vi "ETPA&SPIRTONE PROGRAM V1.vi"() -> ()   [LabVIEW 2024]
uses:
  <vilib>/Instr/_visa.llb/VISA Find Search Mode.ctl
  <vilib>/Instr/_visa.llb/VISA Open Access Mode.ctl
panel:
  in  "PMT counts for average":i32
  out "PMT counts for average":i32
  out "PRESENT MULTIMETER AVERAGE":dbl(graph)
  out "multimeter counts for average":i32
  in  "multimeter counts for average":i32
  out "Multimeter Connecteion status":string
  out "error out 2":errorcluster
  in  "error in (no error)":errorcluster
  out "Monochromator Connecteion status":string
  in  "Close Shutter":bool
  in  "Open Shutter":bool
  out "PRESENT - COUNTER Averaged":dbl(graph)
  in  "Number of Measuments per average PMT WAVESCAN":i32
  out "Number of Measuments per average PMT WAVESCAN":i32
  in  "Monochromator":refnum<visa-resource-name>
  in  "Step Size (nm)":dbl
  in  "End W/L (nm)":dbl
  in  "Start W/L (nm)":dbl
  out "Present Monochromator":dbl(graph)
  out "SHUTTER STATUS":string="SHUTTER O"
  in  "Go scan":bool
  in  "Stop WAVE":bool
  in  "number of measurements":i32
  out "number of measurements":i32
  out "break time ms 2":u32=100
  out "Collection Time 2":u32=1000
  out "Function (1: AC Volts)\nFunction(0: DC Volts)":u16=1
  out "counter  2":tag="Dev1/ctr0"
  out "source  2":tag="/Dev1/PFI14"
  in  "VISA resource name mulitmeter":refnum<visa-resource-name>
  in  "DEFAULT?":bool
  in  "Collection Time":u32
  in  "Label?":bool
  in  "Wavescan?":bool
  in  "file path (dialog if empty)":path
  in  "?":bool
  out "PRESENT - COUNTER":dbl(graph)
  out "PRESENT - Multimeter":dbl(graph)
  in  "Function (1: AC Volts)\nFunction(0: DC Volts)":u16
  in  "break time ms":u32
  in  "source":tag
  in  "counter":tag
  out "Current Trial -Multimeter":dbl(graph)
  out "Current Trial - Singles Photon Count Rate":dbl(graph)
  in  "speed of taking measurments":u32
  # "Default Settings"
  # "CTR0"
  # "USB0"
  # "PFI14"
  # "Not Default Settings"
  # "PLEASE PUT (\".csv\") at the end of your path"
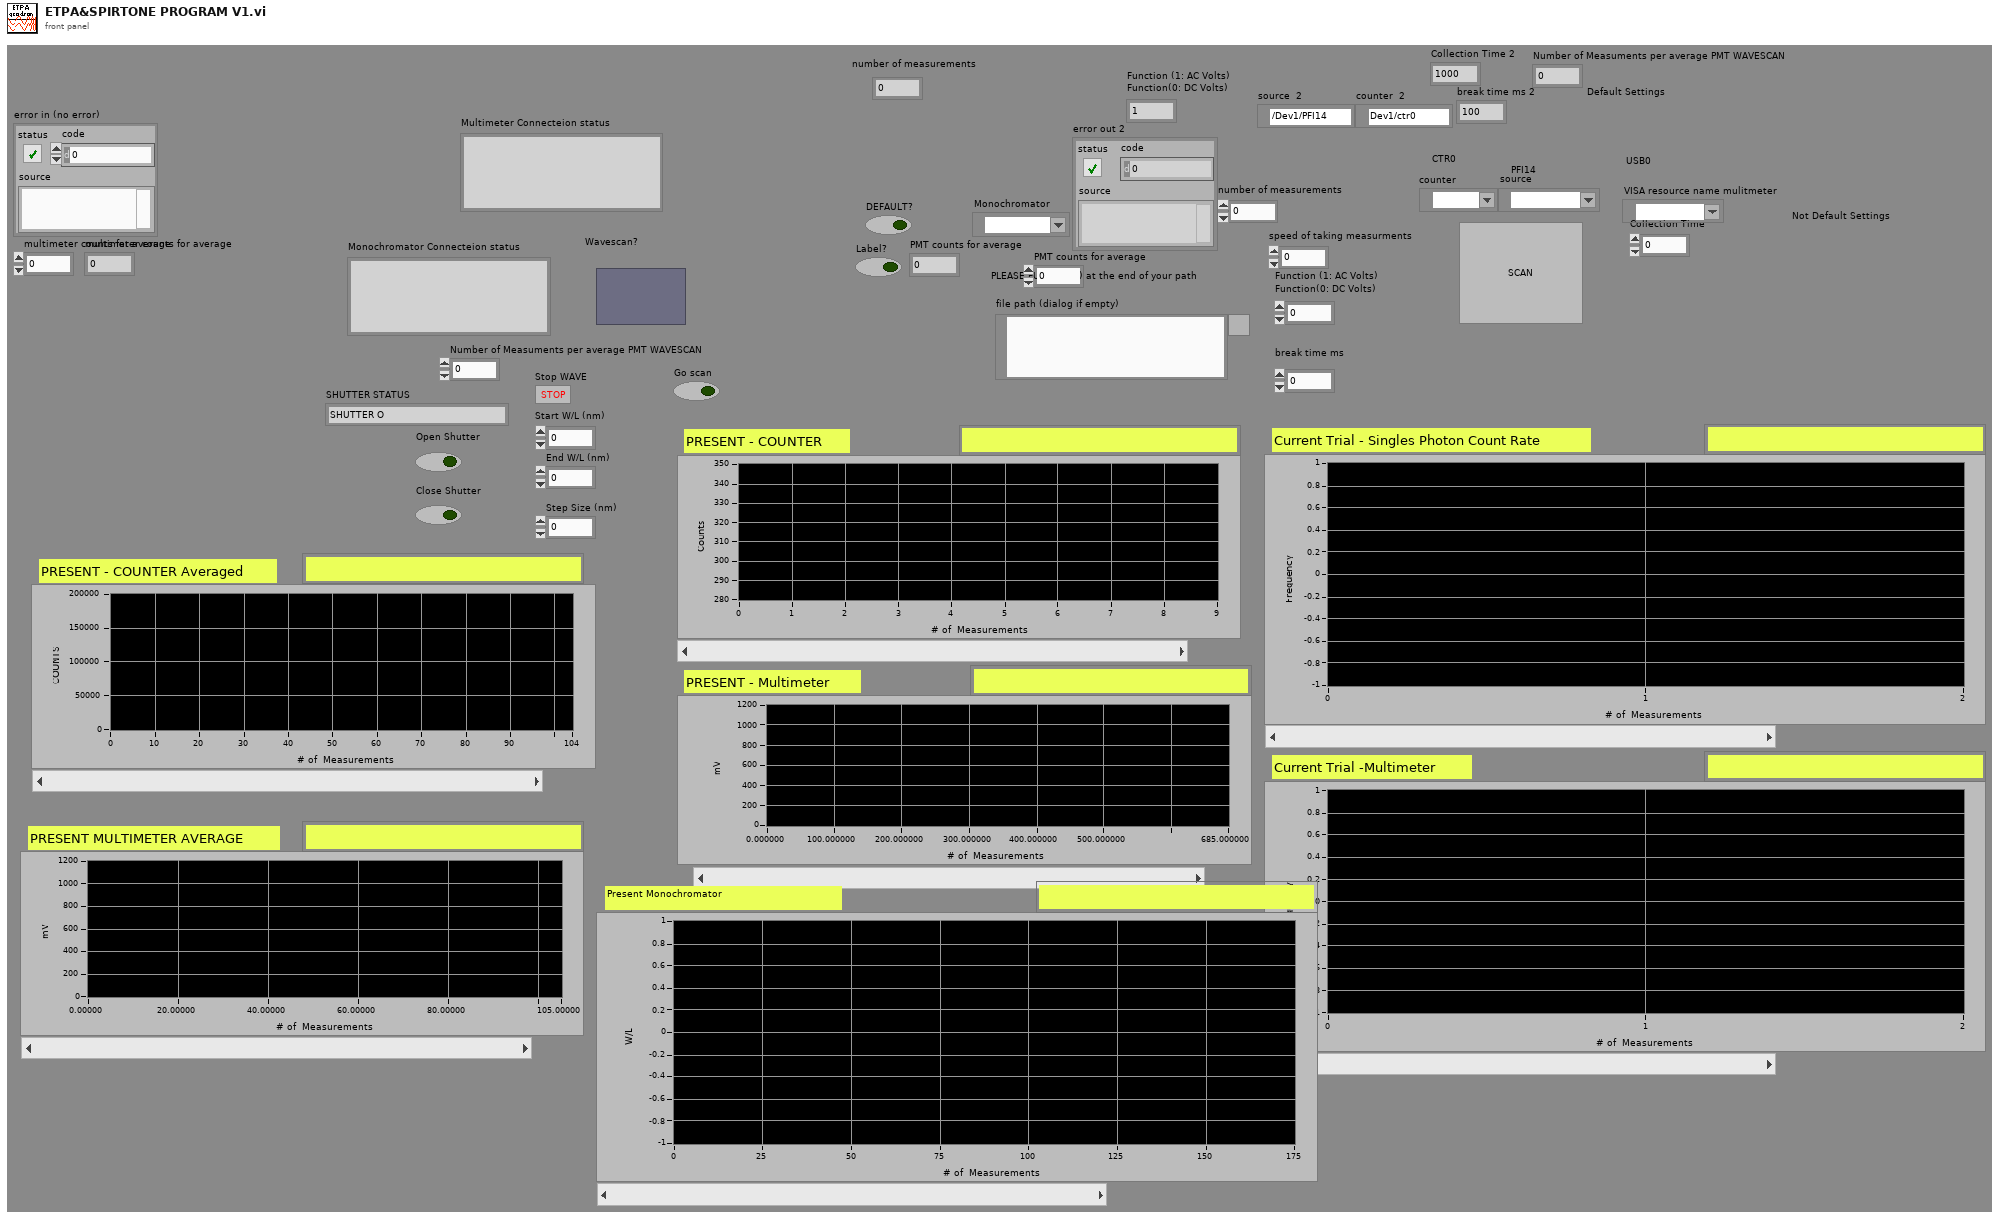
[diagram p1: front panel]
types:
  T1 = typedef "VISA Find Search Mode.ctl" = u32
  T2 = typedef "VISA Open Access Mode.ctl" = u32
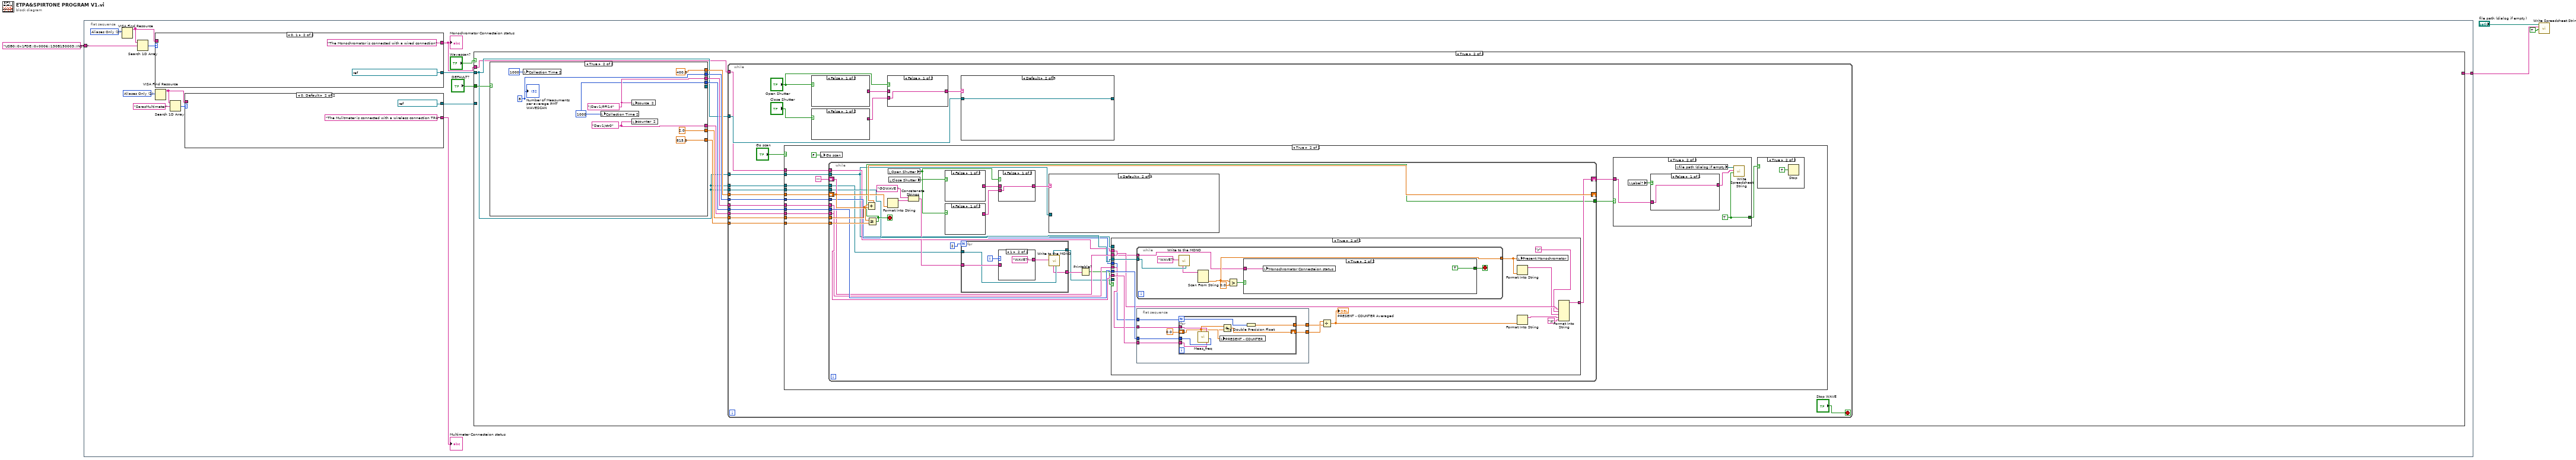
[diagram p0: block diagram]
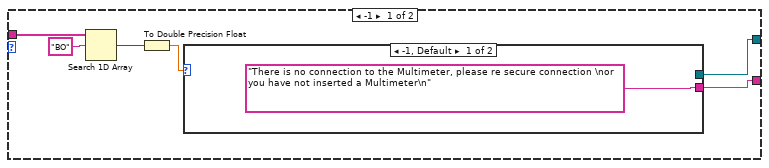
[diagram p2: hidden frame]
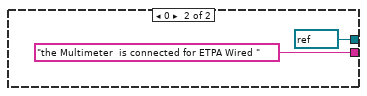
[diagram p3: hidden frame]
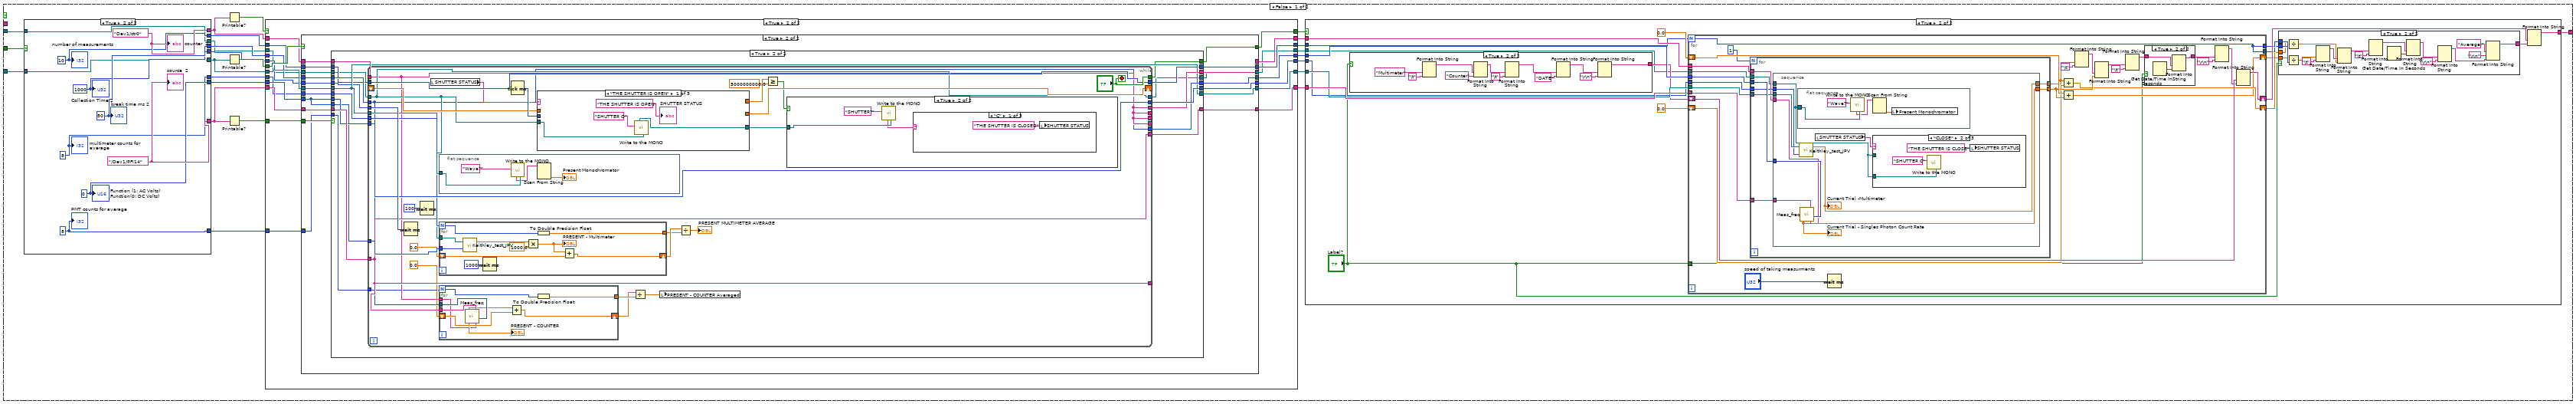
[diagram p4: hidden frame]
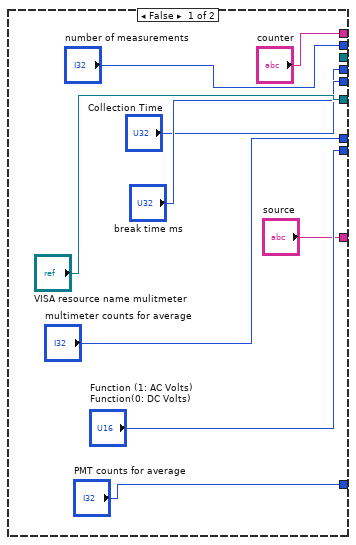
[diagram p5: hidden frame]
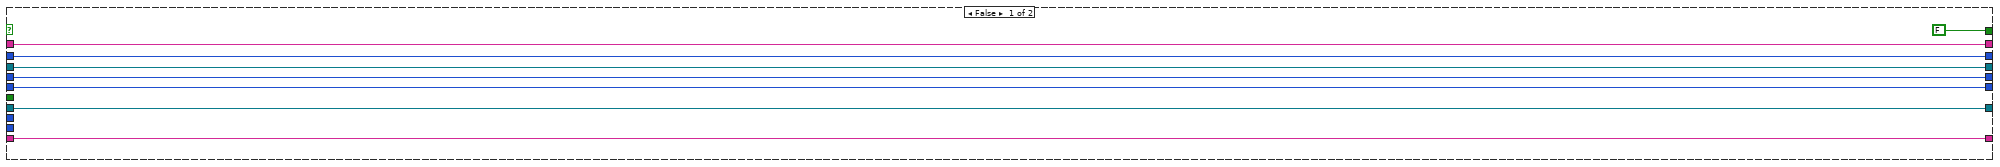
[diagram p6: hidden frame]
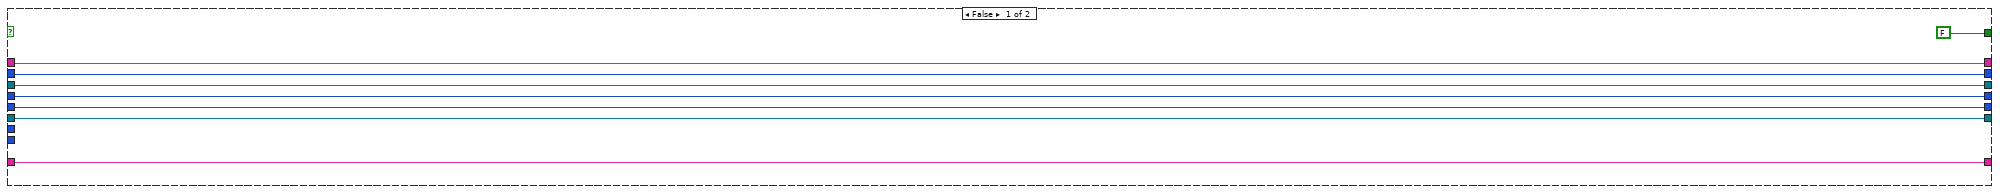
[diagram p7: hidden frame]
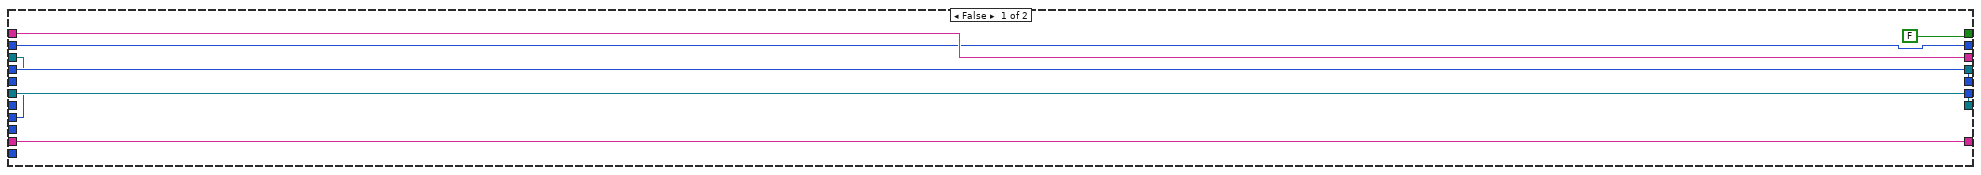
[diagram p8: hidden frame]
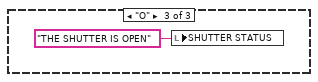
[diagram p11: hidden frame]
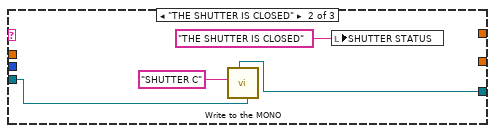
[diagram p12: hidden frame]
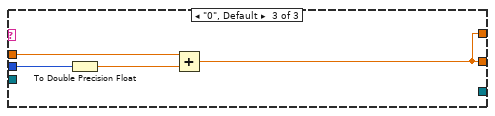
[diagram p13: hidden frame]
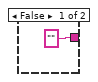
[diagram p14: hidden frame]
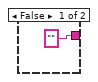
[diagram p15: hidden frame]
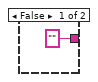
[diagram p16: hidden frame]
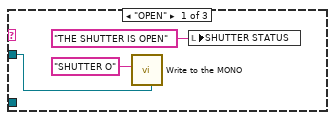
[diagram p18: hidden frame]
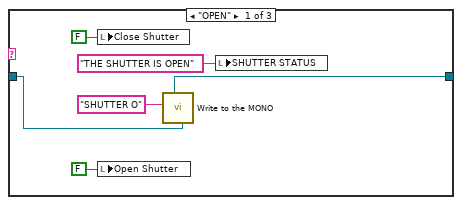
[diagram p20: hidden frame]
diagram:
  n1 = flat-sequence {
    tunnel: [w17] -> w2
    tunnel: "USB0::0x1FDE::0x0006::130B150003::INSTR" ("element") -> [w13]
    frame #0 {
      w10 = T1 2 items=["Canonical Names Only"=0, "Aliases Only"=2, "Include Matching Aliases"=3, "Include All Aliases"=4] ("Search Mode")
      w16 = T1 2 items=["Canonical Names Only"=0, "Aliases Only"=2, "Include Matching Aliases"=3, "Include All Aliases"=4] ("Search Mode")
      n2 = VISA Find Resource(10:w16) -> (3:w15:string[])  [unwired: 2 in, 2 out]
      n3 = Search 1D Array(1D array=w15, element=w13) -> (index of element=w12:i32)  [unwired: 1 in]
      n4 = case shown="0, 1" w12 {
        tunnel: [w523 refnum<visa-resource-name> "USB0::0x1FDE::0x0006::130B150003::INSTR" ("VISA resource name mulitmeter")] -> w14
        tunnel: w15 -> [w525 _]
        tunnel: [w522 "The Monochromator is connected with a wired connection"] -> w11
        frame -1, Default {
          n5 = Search 1D Array(1D array=w525, element="remote130Bmonochromator") -> (index of element=w521:i32)  [unwired: 1 in]
          n6 = To Double Precision Float(number=w521) -> (double precision float=w520:dbl)
          n7 = case shown="-1, Default" w520 {
            tunnel: [_ refnum<visa-resource-name> "USB0::0x1FDE::0x0006::130B150003::INSTR" ("VISA resource name mulitmeter")] -> w523
            tunnel: ["There is no connection to the monochromator, please re secure connection \nor you have not inserted a 130B cornerstone monochromator\n" "the Monochromator is connected romotely"] -> w522
            frame -1, Default {
            }
            frame 0..3 {
            }
          }
        }
        frame 0, 1 {
        }
      }
      "Monochromator Connecteion status" <- w11
      n8 = VISA Find Resource(10:w10) -> (3:w9:string[])  [unwired: 2 in, 2 out]
      n9 = Search 1D Array(1D array=w9, element="SarasMultimeter") -> (index of element=w7:i32)  [unwired: 1 in]
      n10 = case shown="0, Default" w7 {
        tunnel: [w23 refnum<visa-resource-name> "sarasMultimeter" ("VISA resource name mulitmeter")] -> w5
        tunnel: w9 -> [w25 _]
        tunnel: [w22 "The Mulitmeter is connected with a wireless connection TPA"] -> w6
        frame -1 {
          n11 = Search 1D Array(1D array=w25, element="BO") -> (index of element=w21:i32)  [unwired: 1 in]
          n12 = To Double Precision Float(number=w21) -> (double precision float=w20:dbl)
          n13 = case shown="-1, Default" w20 {
            tunnel: [_ refnum<visa-resource-name> "BO" ("VISA resource name mulitmeter")] -> w23
            tunnel: ["There is no connection to the Multimeter, please re secure connection \nor you have not inserted a Multimeter\n" "the Multimeter  is connected for ETPA Wired "] -> w22
            frame -1, Default {
            }
            frame 0 {
            }
          }
        }
        frame 0, Default {
        }
      }
      "Multimeter Connecteion status" <- w6
      n14 = case shown="True" "Wavescan?" {
        tunnel: "DEFAULT?" -> [w40 w340]
        tunnel: [w35 _] -> w17
        tunnel: w14 -> [w34 w332]
        tunnel: w11 -> [_ w331]
        tunnel: w5 -> [w33 _]
        frame False {
          n15 = case shown="True" w40 {
            tunnel: ["VISA resource name mulitmeter" w68] -> w46
            tunnel: ["break time ms" w74] -> w45
            tunnel: ["Collection Time" w73] -> w44
            tunnel: ["Function (1: AC Volts)\nFunction(0: DC Volts)" w67] -> w43
            tunnel: ["source" w72] -> w42
            tunnel: ["counter" w71] -> w41
            tunnel: ["number of measurements" w70] -> w38
            tunnel: [_ w69] -> w37
            tunnel: w34 -> [_ w69]
            tunnel: w33 -> [_ w68]
            tunnel: ["multimeter counts for average" w66] -> w32
            tunnel: ["PMT counts for average" w65] -> w31
            frame False {
            }
            frame True {
              w65 = 8 ("PMT counts for average")
              w66 = 8 ("Numeric 2")
              w67 = u16 0 ("Function (1: AC Volts)\nFunction(0: DC Volts)")
              w70 = 10
              w71 = tag "Dev1/ctr0" ("counter")
              w72 = tag "/Dev1/PFI14" ("source")
              w73 = u32 1000 ("Collection Time")
              w74 = u32 50 ("break time ms")
              "source  2" <- w72
              "counter  2" <- w71
              "Function (1: AC Volts)\nFunction(0: DC Volts)" <- w67
              "Collection Time 2" <- w73
              "break time ms 2" <- w74
              "number of measurements" <- w70
              "multimeter counts for average" <- w66
              "PMT counts for average" <- w65
            }
          }
          n16 = Printable?(1:w41) -> (0:w49:bool)
          n17 = Printable?(1:w46) -> (0:w48:bool)
          n18 = Printable?(1:w42) -> (0:w47:bool)
          n19 = case shown="True" w49 {
            tunnel: w48 -> [_ w102]
            tunnel: w47 -> [_ w101]
            tunnel: w41 -> [w80 w100]
            tunnel: w46 -> [w78 w99]
            tunnel: w42 -> [w81 w98]
            tunnel: w45 -> [w79 w97]
            tunnel: w43 -> [_ w96]
            tunnel: [w81 w95] -> w55
            tunnel: [w78 w94] -> w54
            tunnel: [w79 w93] -> w53
            tunnel: [w80 w92] -> w52
            tunnel: [FALSE w91] -> w51
            tunnel: [w77 w90] -> w50
            tunnel: w44 -> [w77 w89]
            tunnel: w38 -> [w76 w88]
            tunnel: [w76 w87] -> w39
            tunnel: w37 -> [w75 w86]
            tunnel: [w75 w85] -> w36
            tunnel: w32 -> [_ w84]
            tunnel: w31 -> [_ w83]
            frame False {
            }
            frame True {
              n20 = case shown="True" w102 {
                tunnel: w101 -> [_ w129]
                tunnel: w100 -> [w108 w128]
                tunnel: w99 -> [w107 w113]
                tunnel: w98 -> [w110 w127]
                tunnel: w97 -> [w109 w126]
                tunnel: w96 -> [_ w125]
                tunnel: [w110 w124] -> w95
                tunnel: [w107 w123] -> w94
                tunnel: [w109 w122] -> w93
                tunnel: [w108 w121] -> w92
                tunnel: [FALSE w120] -> w91
                tunnel: [w105 w119] -> w90
                tunnel: w89 -> [w105 w118]
                tunnel: w88 -> [w104 w117]
                tunnel: [w104 w116] -> w87
                tunnel: w86 -> [w103 w115]
                tunnel: [w103 w114] -> w85
                tunnel: w84 -> [_ w112]
                tunnel: w83 -> [_ w111]
                frame False {
                }
                frame True {
                  n21 = case shown="True" w129 {
                    tunnel: [w136 w150] -> w124
                    tunnel: [w137 w149] -> w123
                    tunnel: [w134 w153] -> w122
                    tunnel: [w135 w151] -> w121
                    tunnel: [FALSE w148] -> w120
                    tunnel: [w132 w152] -> w119
                    tunnel: w128 -> [w135 w154]
                    tunnel: w113 -> [w137 w149]
                    tunnel: w127 -> [w136 w155]
                    tunnel: w126 -> [_ w147]
                    tunnel: w125 -> [w134 w146]
                    tunnel: w125 -> [_ w145]
                    tunnel: w118 -> [w132 w144]
                    tunnel: w117 -> [w131 w143]
                    tunnel: [w131 w142] -> w116
                    tunnel: w115 -> [w130 w141]
                    tunnel: [w130 w140] -> w114
                    tunnel: w112 -> [_ w139]
                    tunnel: w111 -> [_ w138]
                    frame False {
                    }
                    frame True {
                      n22 = while {
                        tunnel: [w182] -> w153
                        tunnel: [w162] -> _
                        tunnel: [w161] -> w152
                        tunnel: [w162] -> _
                        tunnel: [w162] -> _
                        tunnel: [w163] -> _
                        tunnel: w149 -> [w166]
                        tunnel: w155 -> [w163]
                        tunnel: w154 -> [w162]
                        tunnel: [w162] -> w151
                        tunnel: [w163] -> w150
                        tunnel: ["?"] -> w148
                        tunnel: w147 -> [w183]
                        tunnel: w146 -> [w182]
                        tunnel: w145 -> [w165]
                        tunnel: w144 -> [w161]
                        tunnel: w143 -> [w181]
                        tunnel: [w181] -> w142
                        shift-right: [w178] -> _
                        shift-left: _ -> [w177]
                        tunnel: w141 -> [w172]
                        tunnel: [w172] -> w140
                        tunnel: w139 -> [w170]
                        tunnel: w138 -> [w158]
                        stop <- "?" stop-if-true
                        n23 = Wait (ms)(milliseconds to wait=w183) -> ()  [unwired: 1 out]
                        n24 = Wait (ms)(milliseconds to wait=u32 100) -> ()  [unwired: 1 out]
                        n25 = local read "SHUTTER STATUS"() -> (w171:string)
                        n26 = flat-sequence {
                          tunnel: w172 -> [w205]
                          frame #0 {
                            n27 = call "Write to the MONO.vi"("MONOCHOMATOR"=w205, "write buffer"="Wave?") -> ("read buffer"=w203:string)  [unwired: 7 in, 2 out]
                            n28 = Scan From String(input string=w203) -> (output 1=→"Present Monochromator":dbl)  [unwired: 4 in, 3 out]
                          }
                        }
                        n29 = for {
                          N: w170 -> [w202]
                          shift-right: [w200] -> w169
                          shift-left: 0.0 -> [w201]
                          tunnel: [w199] -> w168
                          tunnel: w166 -> [w198]
                          tunnel: w165 -> [w197]
                          n30 = call "Keithley_test_JPV.vi"("Function (0: DC Volts)"=w197, "VISA resource name"=w198) -> ("Measurement"=w195:dbl)  [unwired: 1 out]
                          n31 = Wait (ms)(milliseconds to wait=u32 1000) -> ()  [unwired: 1 out]
                          n32 = Multiply(x=w195, y=1000.0) -> (x*y=w193:dbl)
                          "PRESENT - Multimeter" <- w193
                          n33 = To Double Precision Float(number=w202) -> (double precision float=w199:dbl)
                          n34 = Add(x=w193, y=w201) -> (x+y=w200:dbl)
                        }
                        n35 = for {
                          N: w158 -> [w187]
                          tunnel: w163 -> [w192]
                          tunnel: w162 -> [w185]
                          tunnel: w161 -> [w191]
                          shift-right: [w188] -> w156
                          shift-left: 0.0 -> [w190]
                          tunnel: [w186] -> w157
                          n36 = call "Meas_freq.vi"("source"=w192, "Time miliseconds"=w191, "counter"=w185) -> (0:w189:dbl)  [unwired: 1 in]
                          "PRESENT - COUNTER" <- w189
                          n37 = Add(x=w189, y=w190) -> (x+y=w188:dbl)
                          n38 = To Double Precision Float(number=w187) -> (double precision float=w186:dbl)
                        }
                        n39 = Tick Count (ms)() -> (millisecond timer value=w179:u32)
                        n40 = case shown="\"THE SHUTTER IS OPEN\"" w171 {
                          tunnel: w179 -> [_ _ w221]
                          tunnel: [_ _ w222] -> w178
                          tunnel: w177 -> [_ _ w223]
                          tunnel: [_ _ w222] -> w175
                          tunnel: [w213 w217 _] -> w173
                          tunnel: w172 -> [w214 w218 _]
                          frame "THE SHUTTER IS OPEN" {
                            n41 = call "Write to the MONO.vi"("MONOCHOMATOR"=w214, "write buffer"="SHUTTER O") -> ("VISA resource name out"=w213:refnum<visa-resource-name>)  [unwired: 7 in, 2 out]
                            "SHUTTER STATUS" <- "THE SHUTTER IS OPEN" ("String")
                          }
                          frame "THE SHUTTER IS CLOSED" {
                            n42 = call "Write to the MONO.vi"("MONOCHOMATOR"=w218, "write buffer"="SHUTTER C") -> ("VISA resource name out"=w217:refnum<visa-resource-name>)  [unwired: 7 in, 2 out]
                            n43 = local write "SHUTTER STATUS"("THE SHUTTER IS CLOSED" ("String")) -> ()
                          }
                          frame "0", Default {
                            n44 = To Double Precision Float(number=w221) -> (double precision float=w220:dbl)
                            n45 = Add(x=w223, y=w220) -> (x+y=w222:dbl)
                          }
                        }
                        n46 = Divide(x=w156, y=w157) -> (x/y=w159:dbl)
                        n47 = local write "PRESENT - COUNTER Averaged"(w159) -> ()
                        n48 = Divide(x=w169, y=w168) -> (x/y=→"PRESENT MULTIMETER AVERAGE":dbl)
                        n49 = Greater Or Equal?(x=w175, y=5000000000.0) -> (x >= y?=w176:bool)
                        n50 = case shown="True" w176 {
                          tunnel: w173 -> [_ w209]
                          frame False {
                          }
                          frame True {
                            n51 = call "Write to the MONO.vi"("MONOCHOMATOR"=w209, "write buffer"="SHUTTER?") -> ("read buffer"=w207:string)  [unwired: 7 in, 2 out]
                            n52 = case shown="\"C\"" w207 {
                              frame "C" {
                                n53 = local write "SHUTTER STATUS"("THE SHUTTER IS CLOSED" ("SHUTTER STATUS")) -> ()
                              }
                              frame Default {
                              }
                              frame "O" {
                                n54 = local write "SHUTTER STATUS"("THE SHUTTER IS OPEN" ("SHUTTER STATUS")) -> ()
                              }
                            }
                          }
                        }
                      }
                    }
                  }
                }
              }
            }
          }
          n55 = case shown="True" w51 {
            tunnel: w50 -> [_ w242]
            tunnel: w55 -> [_ w241]
            tunnel: w54 -> [_ w240]
            tunnel: w53 -> [_ w239]
            tunnel: w52 -> [_ w238]
            tunnel: w39 -> [_ w227]
            tunnel: ["" w226] -> w35
            tunnel: w36 -> [_ w225]
            frame False {
            }
            frame True {
              n56 = case shown="True" "Label?" {
                tunnel: ["" w249] -> w237
                frame False {
                }
                frame True {
                  n57 = Format Into String("Multimeter" ("input 2"), "\t") -> (resulting string=w253:string)  [unwired: 3 in, 1 out]
                  n58 = Format Into String(w253, "Counter" ("input 2")) -> (resulting string=w248:string)  [unwired: 3 in, 1 out]
                  n59 = Format Into String(w248, "\t") -> (resulting string=w246:string)  [unwired: 3 in, 1 out]
                  n60 = Format Into String(w246, "DATE" ("input 2")) -> (resulting string=w245:string)  [unwired: 3 in, 1 out]
                  n61 = Format Into String(w245, "\r\n") -> (resulting string=w249:string)  [unwired: 3 in, 1 out]
                }
              }
              n62 = for {
                N: w227 -> [w292]
                tunnel: w242 -> [w299]
                tunnel: w241 -> [w298]
                tunnel: w240 -> [w297]
                tunnel: w239 -> [w296]
                tunnel: w238 -> [w295]
                shift-right: [w293] -> w236
                shift-left: w237 -> [w294]
                shift-right: [w277] -> w229
                shift-left: 0.0 -> [w282]
                shift-right: [w278] -> w231
                shift-left: 0.0 -> [w279]
                tunnel: [w292] -> w230
                tunnel: [w292] -> w232
                tunnel: "Label?" -> [w276]
                tunnel: w225 -> [w274]
                n63 = for {
                  N: 1 -> [_]
                  tunnel: w299 -> [w311]
                  tunnel: w298 -> [w310]
                  tunnel: w297 -> [w309]
                  tunnel: w296 -> [w308]
                  tunnel: w295 -> [w307]
                  tunnel: [w306] -> w280
                  tunnel: [w305] -> w281
                  tunnel: w274 -> [w304]
                  n64 = stacked-sequence {
                    tunnel: w311 -> [w320]
                    tunnel: w310 -> [w319]
                    tunnel: w309 -> [w318]
                    tunnel: w308 -> [w317]
                    tunnel: w307 -> [w312]
                    tunnel: [w316] -> w306
                    tunnel: [w315] -> w305
                    tunnel: w304 -> [w313]
                    frame #0 {
                      n65 = flat-sequence {
                        tunnel: w313 -> [w323]
                        frame #0 {
                          n66 = call "Write to the MONO.vi"("MONOCHOMATOR"=w323, "write buffer"="Wave?") -> ("read buffer"=w321:string)  [unwired: 7 in, 2 out]
                          n67 = Scan From String(input string=w321) -> (output 1=w324:dbl)  [unwired: 4 in, 3 out]
                          n68 = local write "Present Monochromator"(w324) -> ()
                        }
                      }
                      n69 = call "Keithley_test_JPV.vi"("Function (0: DC Volts)"=w317, "VISA resource name"=w318) -> ("Measurement"=w316:dbl)  [unwired: 1 out]
                      "Current Trial -Multimeter" <- w316
                      n70 = call "Meas_freq.vi"("source"=w319, "Time miliseconds"=w320, "counter"=w312) -> (0:w315:dbl)  [unwired: 1 in]
                      "Current Trial - Singles Photon Count Rate" <- w315
                      n71 = local read "SHUTTER STATUS"() -> (w314:string)
                      n72 = case shown="\"CLOSE\"" w314 {
                        tunnel: w313 -> [w326 _ _]
                        tunnel: w313 -> [_ w329 _]
                        frame "OPEN" {
                          n73 = call "Write to the MONO.vi"("MONOCHOMATOR"=w326, "write buffer"="SHUTTER O") -> ()  [unwired: 7 in, 3 out]
                          n74 = local write "SHUTTER STATUS"("THE SHUTTER IS OPEN" ("String")) -> ()
                        }
                        frame "CLOSE" {
                          n75 = call "Write to the MONO.vi"("MONOCHOMATOR"=w329, "write buffer"="SHUTTER C") -> ()  [unwired: 7 in, 3 out]
                          n76 = local write "SHUTTER STATUS"("THE SHUTTER IS CLOSE" ("String")) -> ()
                        }
                        frame "0", Default {
                        }
                      }
                    }
                  }
                }
                n77 = Wait (ms)(milliseconds to wait="speed of taking measurments") -> ()  [unwired: 1 out]
                n78 = Add(x=w280, y=w279) -> (x+y=w278:dbl)
                n79 = Add(x=w282, y=w281) -> (x+y=w277:dbl)
                n80 = Format Into String(w280, "\t") -> (resulting string=w286:string)  [unwired: 3 in, 1 out]
                n81 = Format Into String(w286, w281) -> (resulting string=w288:string)  [unwired: 3 in, 1 out]
                n82 = Format Into String(w288, "\t") -> (resulting string=w289:string)  [unwired: 3 in, 1 out]
                n83 = case shown="True" w276 {
                  tunnel: [w300 w303] -> w290
                  tunnel: w289 -> [w300 w302]
                  frame False {
                  }
                  frame True {
                    n84 = Get Date/Time In Seconds() -> (seconds since 1Jan1904=w301:timestamp)
                    n85 = Format Into String(w302, w301) -> (resulting string=w303:string)  [unwired: 3 in, 1 out]
                  }
                }
                n86 = Format Into String(w290, "\r\n") -> (resulting string=w287:string)  [unwired: 3 in, 1 out]
                n87 = Format Into String(w294, w287) -> (resulting string=w293:string)  [unwired: 3 in, 1 out]
              }
              n88 = case shown="True" "Label?" {
                tunnel: ["" w267] -> w233
                tunnel: w232 -> [_ w261]
                tunnel: w231 -> [_ w260]
                tunnel: w230 -> [_ w258]
                tunnel: w229 -> [_ w257]
                frame False {
                }
                frame True {
                  n89 = Divide(x=w257, y=w258) -> (x/y=w256:dbl)
                  n90 = Divide(x=w260, y=w261) -> (x/y=w259:dbl)
                  n91 = Format Into String(w259, "\t") -> (resulting string=w266:string)  [unwired: 3 in, 1 out]
                  n92 = Format Into String(w266, w256) -> (resulting string=w265:string)  [unwired: 3 in, 1 out]
                  n93 = Format Into String(w265, "\t") -> (resulting string=w262:string)  [unwired: 3 in, 1 out]
                  n94 = Get Date/Time In Seconds() -> (seconds since 1Jan1904=w271:timestamp)
                  n95 = Format Into String(w262, w271) -> (resulting string=w273:string)  [unwired: 3 in, 1 out]
                  n96 = Format Into String(w273, "\r\n") -> (resulting string=w268:string)  [unwired: 3 in, 1 out]
                  n97 = Format Into String("Average:" ("input 4"), "\r\n", w268) -> (resulting string=w267:string)  [unwired: 3 in, 1 out]
                }
              }
              n98 = Format Into String(w236, w233) -> (resulting string=w226:string)  [unwired: 3 in, 1 out]
            }
          }
        }
        frame True {
          n99 = case shown="True" w340 {
            tunnel: ["End W/L (nm)" 815.0 ("End W/L (nm)")] -> w339
            tunnel: ["Start W/L (nm)" 400.0 ("Start W/L (nm)")] -> w338
            tunnel: ["Step Size (nm)" 2.0 ("Step Size (nm)")] -> w337
            tunnel: [w506 w512] -> w336
            tunnel: [w507 w516] -> w335
            tunnel: [w508 w515] -> w334
            tunnel: ["Monochromator" _] -> _
            tunnel: ["Number of Measuments per average PMT WAVESCAN" w513] -> w333
            frame False {
              n100 = local read "Collection Time"() -> (w506:u32)
              n101 = local read "counter"() -> (w507:tag)
              n102 = local read "source"() -> (w508:tag)
            }
            frame True {
              w512 = u32 1000 ("Collection Time")
              w513 = 8
              w516 = tag "Dev1/ctr0" ("counter")
              w515 = tag "/Dev1/PFI14" ("source")
              n103 = local write "Collection Time 2"(u32 1000 ("Collection Time")) -> ()
              n104 = local write "Collection Time 2"(w512) -> ()
              n105 = local write "source  2"(w515) -> ()
              n106 = local write "counter  2"(w516) -> ()
              "Number of Measuments per average PMT WAVESCAN" <- w513
            }
          }
          n107 = while {
            tunnel: w339 -> [w357]
            tunnel: w338 -> [w356]
            tunnel: w337 -> [w355]
            tunnel: w336 -> [w354]
            tunnel: w335 -> [w353]
            tunnel: w334 -> [w352]
            tunnel: w333 -> [w351]
            tunnel: w332 -> [w345]
            tunnel: w332 -> [w344]
            tunnel: w332 -> [w343]
            tunnel: w332 -> [w342]
            tunnel: w331 -> [w341]
            stop <- "Stop WAVE" stop-if-true
            n108 = case shown="True" "Go scan" {
              tunnel: w357 -> [_ w392]
              tunnel: w356 -> [_ w391]
              tunnel: w355 -> [_ w390]
              tunnel: w354 -> [_ w389]
              tunnel: w353 -> [_ w388]
              tunnel: w352 -> [_ w387]
              tunnel: w345 -> [_ w386]
              tunnel: w344 -> [_ w385]
              tunnel: w351 -> [_ w383]
              tunnel: w343 -> [_ w382]
              tunnel: w341 -> [_ w377]
              frame False {
              }
              frame True {
                n109 = local write "Go scan"(FALSE) -> ()
                n110 = while {
                  tunnel: w392 -> [w428]
                  shift-right: [w429] -> _
                  shift-left: w391 -> [w427]
                  tunnel: w390 -> [w430]
                  tunnel: w389 -> [w426]
                  tunnel: w388 -> [w425]
                  tunnel: w387 -> [w424]
                  shift-right: [w423] -> w381
                  shift-left: "" -> [w421]
                  tunnel: w386 -> [w408]
                  tunnel: w385 -> [w420]
                  tunnel: [w422] -> w384
                  tunnel: w383 -> [w419]
                  tunnel: w382 -> [w407]
                  tunnel: w377 -> [w412]
                  stop <- w422 stop-if-true
                  n111 = Add(x=w430, y=w427) -> (x+y=w429:dbl)
                  n112 = Greater Or Equal?(x=w427, y=w428) -> (x >= y?=w422:bool)
                  n113 = Format Into String(w427) -> (resulting string=w432:string)  [unwired: 3 in, 1 out]
                  n114 = local read "Open Shutter"() -> (w413:bool)
                  n115 = local read "Close Shutter"() -> (w414:bool)
                  n116 = Concatenate Strings("GOWAVE ", w432) -> (w418:string)
                  n117 = case shown="False" w413 {
                    tunnel: [_ "OPEN"] -> w416
                    frame False {
                    }
                    frame True {
                    }
                  }
                  n118 = case shown="False" w414 {
                    tunnel: [_ "CLOSE"] -> w417
                    frame False {
                    }
                    frame True {
                    }
                  }
                  n119 = for {
                    N: 2 -> [_]
                    tunnel: w418 -> [w438]
                    tunnel: [w433] -> w410
                    tunnel: w408 -> [w436]
                    tunnel: [w435] -> w406
                    i -> [w437]
                    n120 = case shown="1" w437 {
                      tunnel: w438 -> [w439 _]
                      tunnel: [w439 "WAVE?"] -> w434
                      frame 0, Default {
                      }
                      frame 1 {
                      }
                    }
                    n121 = call "Write to the MONO.vi"("MONOCHOMATOR"=w436, "write buffer"=w434) -> ("read buffer"=w433:string, "VISA resource name out"=w435:refnum<visa-resource-name>)  [unwired: 7 in, 1 out]
                  }
                  n122 = case shown="False" w413 {
                    tunnel: [w451 w452] -> w415
                    tunnel: w417 -> [w451 _]
                    tunnel: w416 -> [_ w452]
                    frame False {
                    }
                    frame True {
                    }
                  }
                  n123 = case shown="Default" w415 {
                    tunnel: w407 -> [w444 _ w449]
                    frame "OPEN" {
                      n124 = local write "Open Shutter"(FALSE) -> ()
                      n125 = local write "Close Shutter"(FALSE) -> ()
                      n126 = call "Write to the MONO.vi"("MONOCHOMATOR"=w444, "write buffer"="SHUTTER O") -> ()  [unwired: 7 in, 3 out]
                      n127 = local write "SHUTTER STATUS"("THE SHUTTER IS OPEN" ("String")) -> ()
                    }
                    frame Default {
                    }
                    frame "CLOSE" {
                      n128 = local write "Open Shutter"(FALSE) -> ()
                      n129 = local write "Close Shutter"(FALSE) -> ()
                      n130 = call "Write to the MONO.vi"("MONOCHOMATOR"=w449, "write buffer"="SHUTTER C") -> ()  [unwired: 7 in, 3 out]
                      n131 = local write "SHUTTER STATUS"("THE SHUTTER IS CLOSED" ("String")) -> ()
                    }
                  }
                  n132 = Printable?(1:w410) -> (0:w409:bool)
                  n133 = case shown="True" w409 {
                    tunnel: w426 -> [_ w475]
                    tunnel: w425 -> [_ w474]
                    tunnel: w424 -> [_ w473]
                    tunnel: [_ w466] -> w423
                    tunnel: w421 -> [_ w467]
                    tunnel: w420 -> [_ w472]
                    tunnel: w419 -> [_ w471]
                    tunnel: w412 -> [_ w461]
                    tunnel: w407 -> [_ _]
                    tunnel: w406 -> [w459 _]
                    frame False {
                      w455 = T2 0 items=["VISA Defaults"=0, "Exclusive Lock"=1, "Load Configured Settings"=4] ("Access Mode")
                      n134 = property class="Instr" props=["TermChar"](reference=w459) -> (reference out=w456:refnum<visa-resource-name>)  [unwired: 1 in, 2 out]
                      n135 = VISA Open(access mode=w455, VISA resource name=w456) -> ()  [unwired: 3 in, 2 out]
                      n136 = VISA Close(VISA resource name=w456, error in (no error)="error in (no error)") -> (error out=→"error out 2":errorcluster)
                    }
                    frame True {
                      n137 = while {
                        tunnel: w472 -> [w498]
                        tunnel: [w495] -> w468
                        tunnel: w461 -> [w494]
                        stop <- w493 stop-if-true
                        n138 = call "Write to the MONO.vi"("MONOCHOMATOR"=w498, "write buffer"="WAVE?") -> ("read buffer"=w491:string)  [unwired: 7 in, 2 out]
                        n139 = Scan From String(input string=w491) -> (output 1=w495:dbl)  [unwired: 4 in, 3 out]
                        n140 = Greater?(x=w495, y=0.0) -> (0:w496:bool)
                        n141 = case shown="True" w496 {
                          tunnel: w494 -> [_ w503]
                          tunnel: [FALSE TRUE] -> w493
                          frame False {
                            n142 = Wait (ms)(milliseconds to wait=u32 500 ("millisecond timer value")) -> ()  [unwired: 1 out]
                            n143 = local write "Monochromator Connecteion status"("Connection was unstable retrying") -> ()
                          }
                          frame True {
                            n144 = local write "Monochromator Connecteion status"(w503) -> ()
                          }
                        }
                      }
                      n145 = flat-sequence {
                        tunnel: w475 -> [w482]
                        tunnel: w474 -> [w481]
                        tunnel: w473 -> [w480]
                        tunnel: w471 -> [w479]
                        tunnel: [w478] -> w470
                        tunnel: [w477] -> w469
                        frame #0 {
                          n146 = for {
                            N: w479 -> [w489]
                            shift-right: [w490] -> w477
                            shift-left: 0.0 -> [w484]
                            tunnel: [w488] -> w478
                            tunnel: w480 -> [w487]
                            tunnel: w481 -> [w483]
                            tunnel: w482 -> [w486]
                            n147 = call "Meas_freq.vi"("source"=w487, "Time miliseconds"=w486, "counter"=w483) -> (0:w485:dbl)  [unwired: 1 in]
                            n148 = local write "PRESENT - COUNTER"(w485) -> ()
                            n149 = Add(x=w485, y=w484) -> (x+y=w490:dbl)
                            n150 = To Double Precision Float(number=w489) -> (double precision float=w488:dbl)
                          }
                        }
                      }
                      n151 = Divide(x=w469, y=w470) -> (x/y=w460:dbl)
                      "PRESENT - COUNTER Averaged" <- w460
                      n152 = local write "Present Monochromator"(w468) -> ()
                      n153 = Format Into String(w468) -> (resulting string=w464:string)  [unwired: 3 in, 1 out]
                      n154 = Format Into String(w460) -> (resulting string=w463:string)  [unwired: 3 in, 1 out]
                      n155 = Format Into String(w467, "\r", w464, w463, "\t") -> (resulting string=w466:string)  [unwired: 3 in, 1 out]
                    }
                  }
                }
                n156 = case shown="True" w384 {
                  tunnel: w381 -> [_ w395]
                  tunnel: [_ w396] -> w379
                  frame False {
                  }
                  frame True {
                    w396 = TRUE ("append to file? (new file:F)")
                    n157 = local read "Label?"() -> (w398:bool)
                    n158 = case shown="False" w398 {
                      tunnel: w395 -> [w399 w401]
                      tunnel: [w399 w400] -> w394
                      frame False {
                      }
                      frame True {
                        n159 = Format Into String("W/L", "\t", "Counts", "\r\n", w401) -> (resulting string=w400:string)  [unwired: 3 in, 1 out]
                      }
                    }
                    n160 = local read "file path (dialog if empty)"() -> (w397:path)
                    n161 = call <vilib>:"Write Spreadsheet String.vi"("append to file? (new file:F)"=w396, "spreadsheet string"=w394, "file path (dialog if empty)"=w397) -> ()  [unwired: 7 in, 2 out]
                  }
                }
                n162 = case shown="True" w379 {
                  frame False {
                  }
                  frame True {
                    n163 = Stop(stop? (T)=TRUE) -> ()
                  }
                }
              }
            }
            n164 = case shown="False" "Open Shutter" {
              tunnel: [_ "OPEN"] -> w348
              frame False {
              }
              frame True {
              }
            }
            n165 = case shown="False" "Close Shutter" {
              tunnel: [_ "CLOSE"] -> w349
              frame False {
              }
              frame True {
              }
            }
            n166 = case shown="False" "Open Shutter" {
              tunnel: [w373 w374] -> w346
              tunnel: w349 -> [w373 _]
              tunnel: w348 -> [_ w374]
              frame False {
              }
              frame True {
              }
            }
            n167 = case shown="Default" w346 {
              tunnel: w342 -> [w364 w366 w371]
              tunnel: [w361 w366 w368] -> _
              frame "OPEN" {
                n168 = local write "Close Shutter"(FALSE) -> ()
                n169 = local write "Open Shutter"(FALSE) -> ()
                n170 = call "Write to the MONO.vi"("MONOCHOMATOR"=w364, "write buffer"="SHUTTER O") -> ("VISA resource name out"=w361:refnum<visa-resource-name>)  [unwired: 7 in, 2 out]
                n171 = local write "SHUTTER STATUS"("THE SHUTTER IS OPEN" ("String")) -> ()
              }
              frame Default {
              }
              frame "CLOSE" {
                n172 = local write "Open Shutter"(FALSE) -> ()
                n173 = local write "Close Shutter"(FALSE) -> ()
                n174 = call "Write to the MONO.vi"("MONOCHOMATOR"=w371, "write buffer"="SHUTTER C") -> ("VISA resource name out"=w368:refnum<visa-resource-name>)  [unwired: 7 in, 2 out]
                n175 = local write "SHUTTER STATUS"("THE SHUTTER IS CLOSED" ("String")) -> ()
              }
            }
          }
        }
      }
    }
  }
  n176 = call <vilib>:"Write Spreadsheet String.vi"("append to file? (new file:F)"=TRUE, "spreadsheet string"=w2, "file path (dialog if empty)"="file path (dialog if empty)") -> ()  [unwired: 7 in, 2 out]
